vi "Handle Last Ack Core.vi"(4 "error in (no error)":errorcluster, 6 "Last Ack":refnum<class "Last Ack.lvclass">, 7 "WebSocket Server Manager in":refnum<class "WebSocket Server Manager.lvclass">) -> (0 "error out":errorcluster, 3 "WebSocket Server Manager out":refnum<class "WebSocket Server Manager.lvclass">)   [LabVIEW 2016, in "WebSocket Actors.lvlib" / "WebSocket Server Manager.lvclass"]
doc: "(<B>Filename</B>: Actor Framework.lvlib:Actor.lvclass:Handle Last Ack Core.vi)\n\nDefines how the caller actor responds to the Last Ack message from a nested actor. The Last Ack message is the final message a nested actor sends to its caller before it shuts down. The message contains information about the final state of the nested actor.\n\nBy default, this method does nothing except return any error the nested actor sent. A descendant class may override this method to define behavior."
uses:
  WebSocket Server Manager.lvclass
  <vilib>/ActorFramework/LastAck/Last Ack.lvclass
  WebSocket Server/WebSocket Server.lvclass
  <vilib>/ActorFramework/LastAck/Last Ack.lvclass/Last Ack.ctl
  WebSocket Server/WebSocket Server.lvclass/WebSocket Server.ctl
  WebSocket Server Manager.lvclass/WebSocket Server Manager.ctl
  WebSocket Server/properties/Read URI.vi
  <vilib>/regexp/Match Regular Expression.xnode
  <vilib>/MGI/Monitored Actor/Monitored Actor/Monitored Actor/Monitored Actor.lvclass
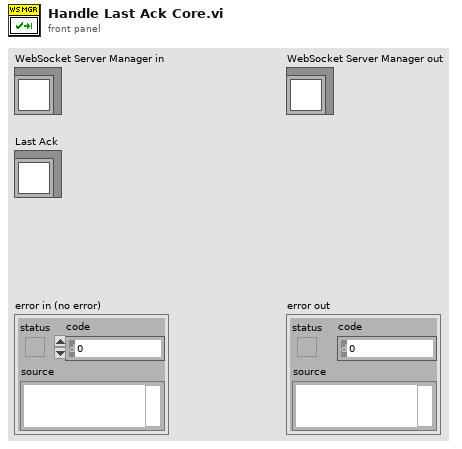
[diagram p1: front panel]
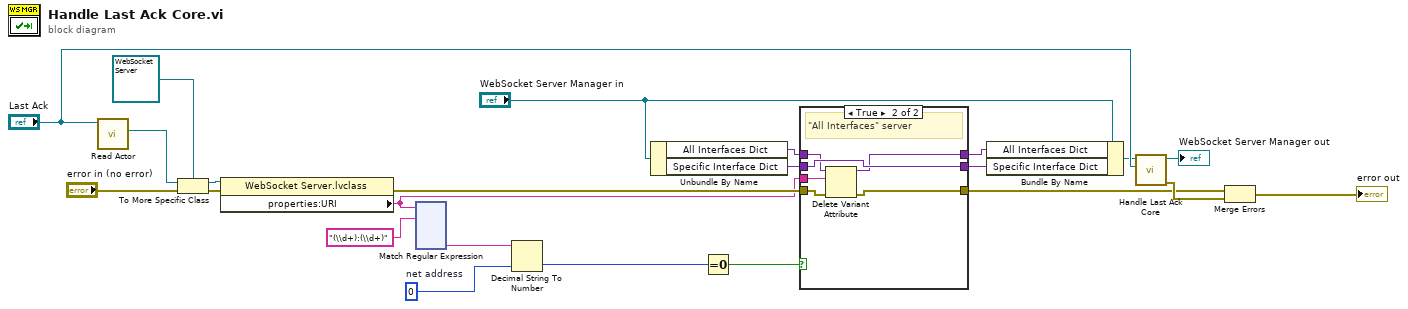
[diagram p0: block diagram]
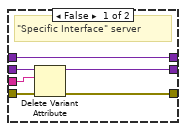
[diagram p2: hidden frame]
diagram:
  w16 = u32 0  # net address
  n1 = call <vilib>:"Read Actor.vi"("Last Ack"="Last Ack") -> ("Actor"=w21:refnum<class "Actor.lvclass">)  [unwired: 10 in]
  n2 = To More Specific Class(target class=refnum<class "WebSocket Server.lvclass"> refnum ("WebSocket Actors.lvlib:WebSocket Server.lvclass"), reference=w21, error in="error in (no error)") -> (specific class reference=w20:refnum<class "WebSocket Server.lvclass">, error out=w5:errorcluster)
  n3 = property class="WebSocket Server.lvclass"(reference=w20, error in=w5) -> (error out=w4:errorcluster, "properties:URI"=w3:string)  [unwired: 1 out]
  n4 = xnode "Match Regular Expression"("input string"=w3, "regular expression"="(\\d+):(\\d+)") -> ("submatch 1"=w17:string)  [unwired: 4 in, 5 out]
  n5 = Decimal String To Number(string=w17, default (0L)=w16) -> (number=w15:u32)  [unwired: 1 in, 1 out]
  n6 = Unbundle By Name("WebSocket Server Manager in") -> ("All Interfaces Dict"=w12:variant, "Specific Interface Dict"=w11:variant)
  n7 = Equal To 0?(x=w15) -> (x = 0?=w14:bool)
  n8 = case shown="True" w14 {
    tunnel: w12 -> [w29 w31]
    tunnel: w11 -> [w28 w35]
    tunnel: [w27 w35] -> w8
    tunnel: [w29 w32] -> w9
    tunnel: w4 -> [w26 w34]
    tunnel: [w25 w33] -> w1
    tunnel: w3 -> [w24 w30]
    frame False {
      # "\"Specific Interface\" server"
      n9 = Delete Variant Attribute(4:w26, 6:w24, 7:w28) -> (0:w25:errorcluster, 3:w27:variant)  [unwired: 1 out]
    }
    frame True {
      # "\"All Interfaces\" server"
      n10 = Delete Variant Attribute(4:w34, 6:w30, 7:w31) -> (0:w33:errorcluster, 3:w32:variant)  [unwired: 1 out]
    }
  }
  n11 = Bundle By Name(cluster="WebSocket Server Manager in", "All Interfaces Dict"=w9, "Specific Interface Dict"=w8) -> (w7:refnum<class "WebSocket Server Manager.lvclass">)
  n12 = call-parent "Handle Last Ack Core.vi"("Last Ack"="Last Ack", "Actor in"=w7) -> ("error out"=w23:errorcluster, "Actor out"=→"WebSocket Server Manager out":refnum<class "WebSocket Server Manager.lvclass">)  [unwired: 4 in]
  n13 = Merge Errors(w1, w23) -> (→"error out":errorcluster)
